vi "Read EnqueuerMap.vi"(8 "error in (no error)":errorcluster, 11 "SuperActor in":refnum<class "SuperActor.lvclass">) -> (0 "error out":errorcluster, 2 "EnqueuerMap":variant, 3 "SuperActor out":refnum<class "SuperActor.lvclass">)   [LabVIEW 2016, in "SuperActor.lvlib" / "SuperActor.lvclass"]
uses:
  SuperActor.lvclass
  SuperActor.lvclass/SuperActor.ctl
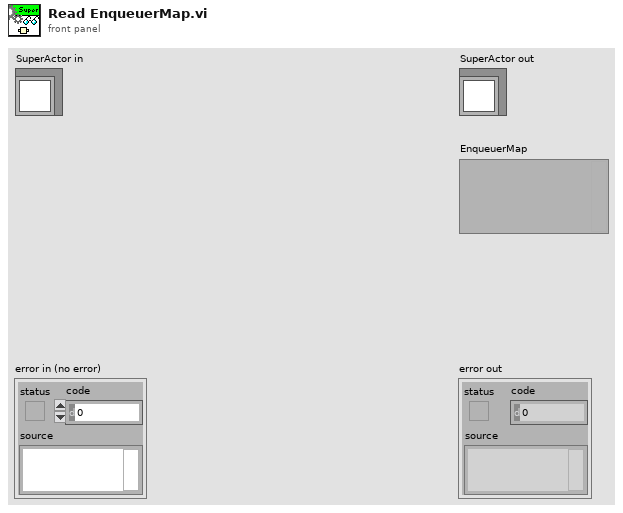
[diagram p1: front panel]
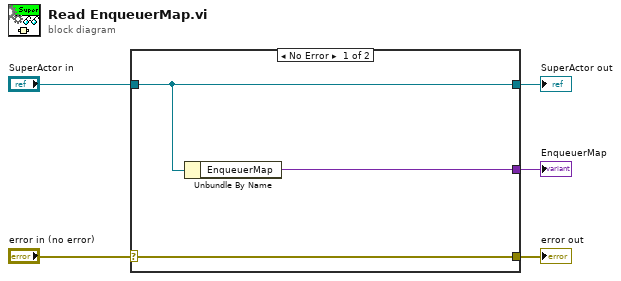
[diagram p0: block diagram]
diagram:
  n1 = case shown="No Error" "error in (no error)" {
    selector: "error in (no error)" -> [w8 w9]
    tunnel: [w8 w9] -> w4
    tunnel: [w7 w10] -> w2
    tunnel: "SuperActor in" -> [w7 w10]
    tunnel: [w6 _] -> w1
    frame No Error {
      n2 = Unbundle By Name(w7) -> ("EnqueuerMap"=w6:variant)
    }
    frame Error {
    }
  }
  "error out" <- w4
  "SuperActor out" <- w2
  "EnqueuerMap" <- w1
